vi "LEDControl.vi"(11 "RobotDriveDevRef 2":T1={"DevStatus"={"status"=FALSE, "code"=0, "source"=""}, "Motors[]"=[], "Square Inputs"=FALSE, "Max Output"=1.0}) -> ()   [LabVIEW 2015]
doc: "LED controls"
uses:
  <vilib>/Rock Robotics/WPI/RobotDrive/WPI_RobotDriveDevRef.ctl
  <vilib>/Rock Robotics/WPI/MotorControl/WPI_MotorControlDeviceRef.ctl
  <vilib>/Rock Robotics/SystemInterfaces/Typedef/FPGA_TypedefDigitalModule.ctl
  <vilib>/Rock Robotics/SystemInterfaces/DIO/FPGA_DIOPWMChannel.ctl
  <vilib>/Rock Robotics/WPI/PWM/WPI_PWMDeadband.ctl
  <vilib>/Rock Robotics/WPI/CAN/Jaguar/SubVIs/WPI_CANJaguar_ControlMode.ctl
  <vilib>/Rock Robotics/WPI/PWM/WPI_PWMTransform_ConPane.ctl
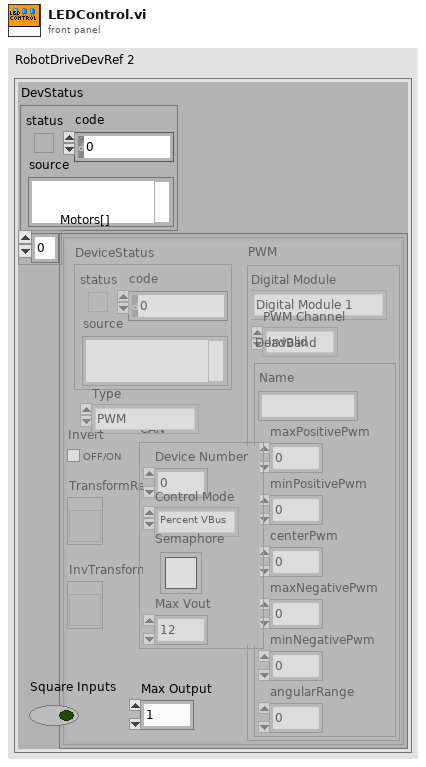
[diagram p1: front panel]
types:
  T1 = typedef "WPI_RobotDriveDevRef.ctl" = cluster{"DevStatus":errorcluster, "Motors[]":T2[], "Square Inputs":bool, "Max Output":dbl}
  T2 = typedef "WPI_MotorControlDeviceRef.ctl" = cluster{"DeviceStatus":errorcluster, "Type":enum16{"PWM", "CAN"}, "PWM":cluster{"Digital Module":T3, "PWM Channel":T4, "DeadBand":T5}, "CAN":cluster{"Device Number":u8, "Control Mode":T6, "Semaphore":T7, "Max Vout":dbl}, "Invert":bool, "TransformRef":T8, "InvTransformRef":T8}
  T3 = typedef "FPGA_TypedefDigitalModule.ctl" = enum16{"Digital Module 1", "Digital Module 2"}
  T4 = typedef "FPGA_DIOPWMChannel.ctl" = enum8{"PWM 1", "PWM 2", "PWM 3", "PWM 4", "PWM 5", "PWM 6", "PWM 7", "PWM 8", "PWM 9", "PWM 10", "Invalid"}
  T5 = typedef "WPI_PWMDeadband.ctl" = cluster{"Name":string, "maxPositivePwm":i32, "minPositivePwm":i32, "centerPwm":i32, "maxNegativePwm":i32, "minNegativePwm":i32, "angularRange":u16}
  T6 = typedef "WPI_CANJaguar_ControlMode.ctl" = enum8{"Percent VBus", "Current", "Speed", "Position", "Voltage"}
  T7 = typedef "Semaphore RefNum" = refnum<k1>
  T8 = typedef "WPI_PWMTransform_ConPane.ctl" = refnum<vi>
  T9 = typedef "WPI_DigitalOutputDevRef.ctl" = cluster{"Digital Module":T3, "DIO Channel":T10, "DevStatus":errorcluster}
  T10 = typedef "FPGA_DIOChannel.ctl" = enum8{"DIO 1", "DIO 2", "DIO 3", "DIO 4", "DIO 5", "DIO 6", "DIO 7", "DIO 8", "DIO 9", "DIO 10", "DIO 11", "DIO 12", "DIO 13", "DIO 14", "Invalid"}
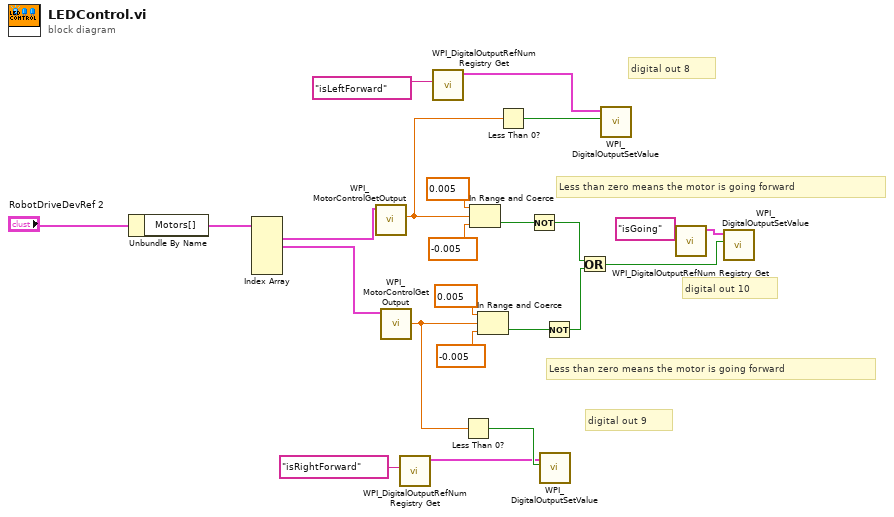
[diagram p0: block diagram]
diagram:
  # "digital out 10"
  # "digital out 9"
  # "digital out 8"
  # "Less than zero means the motor is going forward"
  # "Less than zero means the motor is going forward"
  n1 = Unbundle By Name("RobotDriveDevRef 2") -> ("Motors[]"=w16:T2[])
  n2 = Index Array(array=w16) -> (element #1=w17:T2, element #2=w21:T2)  [unwired: 5 in, 3 out]
  n3 = call <vilib>:"WPI_MotorControlGetOutput.vi"("MotorControlDevRef"=w17) -> ("Output"=w8:dbl)  [unwired: 8 in, 2 out]
  n4 = call <vilib>:"WPI_MotorControlGetOutput.vi"("MotorControlDevRef"=w21) -> ("Output"=w1:dbl)  [unwired: 8 in, 2 out]
  n5 = call <vilib>:"WPI_DigitalOutputRefNum Registry Get.vi"("refnum name"="isRightForward") -> ("DigitalOutputDevRef"=w19:T9)  [unwired: 9 in, 1 out]
  n6 = call <vilib>:"WPI_DigitalOutputRefNum Registry Get.vi"("refnum name"="isLeftForward") -> ("DigitalOutputDevRef"=w20:T9)  [unwired: 9 in, 1 out]
  n7 = Less Than 0?(x=w1) -> (x < 0?=w23:bool)
  n8 = In Range and Coerce(upper limit=0.005, x=w8, lower limit=-0.005) -> (In Range?=w9:bool)  [unwired: 1 out]
  n9 = In Range and Coerce(upper limit=0.005, x=w1, lower limit=-0.005) -> (In Range?=w3:bool)  [unwired: 1 out]
  n10 = Less Than 0?(x=w8) -> (x < 0?=w7:bool)
  n11 = Not(x=w9) -> (.not. x?=w6:bool)
  n12 = call <vilib>:"WPI_DigitalOutputSetValue.vi"("Value"=w23, "DigitalOutputDevRef"=w19) -> ()  [unwired: 8 in, 2 out]
  n13 = Not(x=w3) -> (.not. x?=w2:bool)
  n14 = Or(x=w6, y=w2) -> (x .or. y?=w22:bool)
  n15 = call <vilib>:"WPI_DigitalOutputSetValue.vi"("Value"=w7, "DigitalOutputDevRef"=w20) -> ()  [unwired: 8 in, 2 out]
  n16 = call <vilib>:"WPI_DigitalOutputRefNum Registry Get.vi"("refnum name"="isGoing") -> ("DigitalOutputDevRef"=w18:T9)  [unwired: 9 in, 1 out]
  n17 = call <vilib>:"WPI_DigitalOutputSetValue.vi"("Value"=w22, "DigitalOutputDevRef"=w18) -> ()  [unwired: 8 in, 2 out]
